vi "Main_backup.vi"() -> ()   [LabVIEW 2019]
uses:
  <vilib>/ptbypt/NI_PtbyPt.lvlib
panel:
  in  "low cutoff freq y":dbl=0.125 format="%0.3f"
  out "Filtered Correction y":dbl format="%0.2f"
  out "Filtered Correction x":dbl format="%0.2f"
  in  "low cutoff freq x":dbl=0.1 format="%#_13g"
  out "Filtered Correction y":dbl(graph)
  out "Filtered Correction x":dbl(graph)
  out "Height":dbl
  out "Motor 4 Correction":dbl
  out "Motor 3 Correction":dbl
  out "Motor 2 Correction":dbl
  out "Motor 1 Correction":dbl
  out "error out":errorcluster
  out "error out 2":errorcluster
  out "error out 5":errorcluster
  out "error out 6":errorcluster
  in  "PID Gains":T1={"Proportional Gain (Kc)"=0.8, "Integral Gain"=0.0, "Derivative Gain"=0.0}
  in  "Initial Motor Power":dbl
  in  "Boolean":bool
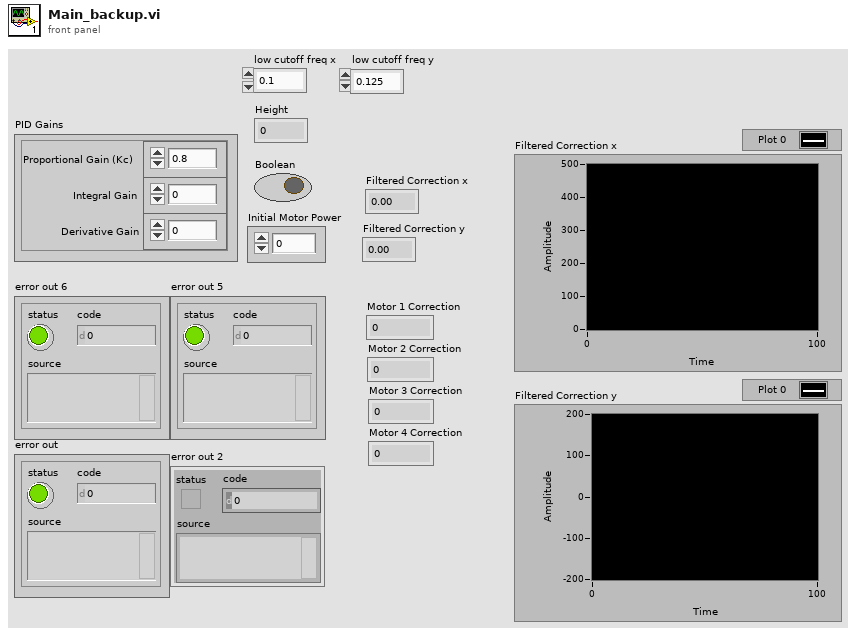
[diagram p1: front panel]
types:
  T1 = cluster{"Proportional Gain (Kc)":dbl, "Integral Gain":dbl, "Derivative Gain":dbl}
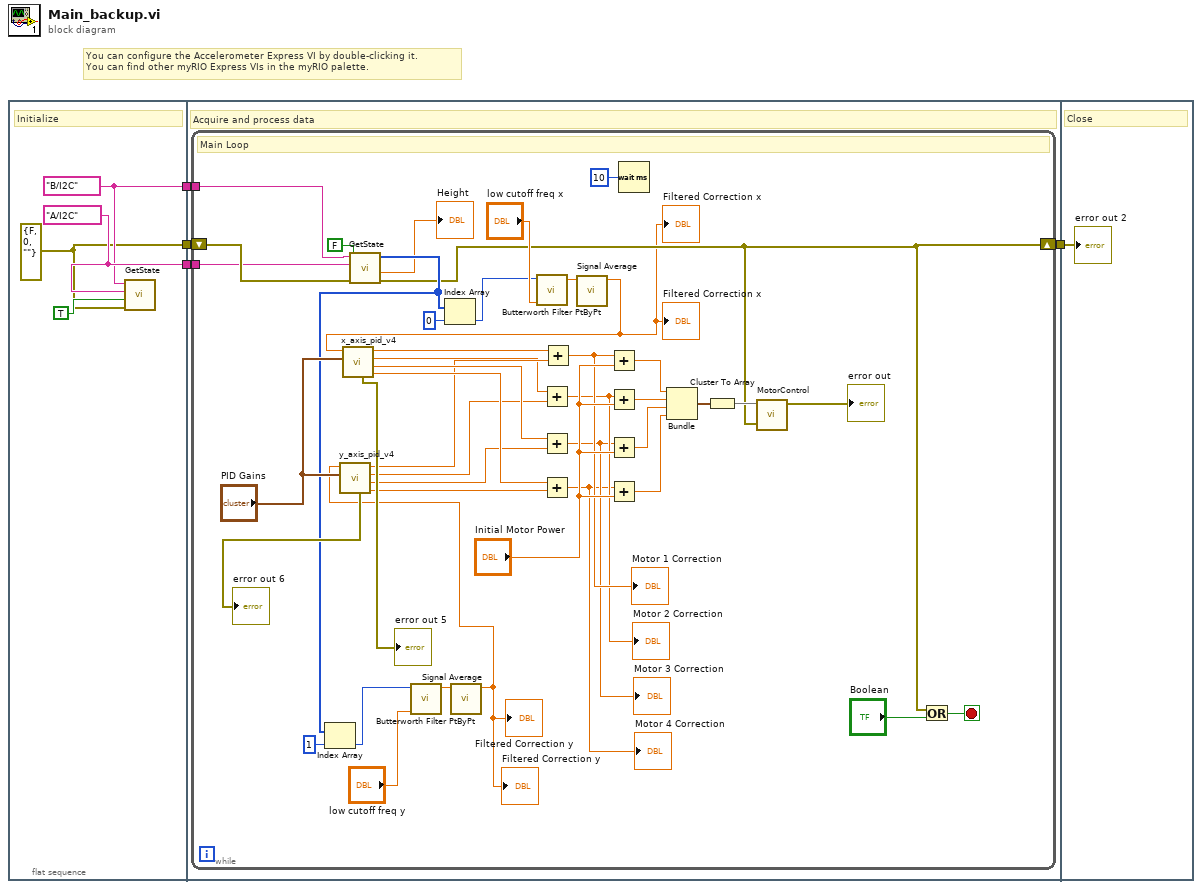
[diagram p0: block diagram]
diagram:
  # "You can configure the Accelerometer Express VI by double-clicking it.\nYou can find other myRIO Express VIs in the myRIO palette."
  n1 = flat-sequence {
    tunnel: [w7] -> w4
    tunnel: [w8] -> w3
    tunnel: [w5] -> w2
    tunnel: [w12] -> w1
    tunnel: w4 -> [w11]
    tunnel: w3 -> [w10]
    tunnel: w2 -> [w9]
    tunnel: w1 -> [w56]
    frame #0 {
      w8 = tag "A/I2C" ("IMU Channel")
      w7 = tag "B/I2C" ("LIDAR Channel")
      w5 = errorcluster {"status"=FALSE, "code"=0, "source"=""} ("error in (no error)")
      # "Initialize"
      n2 = call "GetState.vi"("error in (no error)"=w5, "Calibrate?"=TRUE, "IMU Channel"=w8, "LIDAR Channel"=w7) -> ()  [unwired: 2 in, 4 out]
    }
    frame #1 {
      # "Acquire and process data"
      n3 = while {
        shift-right: [w23] -> w12
        shift-left: w9 -> [w54]
        tunnel: w11 -> [w52]
        tunnel: w10 -> [w51]
        stop <- w55 stop-if-true
        # "Main Loop"
        n4 = call "GetState.vi"("error in (no error)"=w54, "Calibrate?"=FALSE, "IMU Channel"=w51, "LIDAR Channel"=w52) -> ("error out"=w23:errorcluster, "Height"=→"Height":dbl, "imu accel"=w34:i16[])  [unwired: 2 in, 1 out]
        n5 = Index Array(array=w34, index=1) -> (element=w35:i16)
        n6 = call <vilib>:"Butterworth Filter PtByPt.vi"("low cutoff freq: fl"="low cutoff freq y", "x"=w35) -> ("Filtered x"=w14:dbl)  [unwired: 7 in, 1 out]
        n7 = Index Array(array=w34, index=0) -> (element=w37:i16)
        n8 = call "Signal Average.vi"("Filtered Correction"=w14) -> ("Average Signal"=w13:dbl)  [unwired: 10 in]
        "Filtered Correction y" <- w13
        "Filtered Correction y" <- w13
        n9 = call "y_axis_pid_v4.vi"("PID Gains"="PID Gains", "Y In"=w13) -> ("Motor 4"=w41:dbl, "Motor 3"=w42:dbl, "Motor 2"=w43:dbl, "Motor 1"=w25:dbl, "error out"=→"error out 6":errorcluster)  [unwired: 5 in]
        n10 = call <vilib>:"Butterworth Filter PtByPt.vi"("low cutoff freq: fl"="low cutoff freq x", "x"=w37) -> ("Filtered x"=w16:dbl)  [unwired: 7 in, 1 out]
        n11 = call "Signal Average.vi"("Filtered Correction"=w16) -> ("Average Signal"=w17:dbl)  [unwired: 10 in]
        "Filtered Correction x" <- w17
        "Filtered Correction x" <- w17
        n12 = call "x_axis_pid_v4.vi"("PID Gains"="PID Gains", "X In"=w17) -> ("Motor 4"=w44:dbl, "Motor 3"=w45:dbl, "Motor 2"=w24:dbl, "Motor 1"=w46:dbl, "error out"=→"error out 5":errorcluster)  [unwired: 5 in]
        n13 = Add(x=w24, y=w43) -> (x+y=w21:dbl)
        "Motor 2 Correction" <- w21
        n14 = Add(x=w45, y=w42) -> (x+y=w20:dbl)
        "Motor 3 Correction" <- w20
        n15 = Add(x=w44, y=w41) -> (x+y=w19:dbl)
        "Motor 4 Correction" <- w19
        n16 = Add(x=w46, y=w25) -> (x+y=w22:dbl)
        "Motor 1 Correction" <- w22
        n17 = Add(x=w22, y="Initial Motor Power") -> (x+y=w31:dbl)
        n18 = Add(x=w21, y="Initial Motor Power") -> (x+y=w30:dbl)
        n19 = Add(x=w20, y="Initial Motor Power") -> (x+y=w29:dbl)
        n20 = Add(x=w19, y="Initial Motor Power") -> (x+y=w28:dbl)
        n21 = Wait (ms)(milliseconds to wait=u32 10) -> ()  [unwired: 1 out]
        n22 = Bundle(w31, w30, w29, w28) -> (w27:cluster{dbl, dbl, dbl, dbl})  [unwired: 1 in]
        n23 = Cluster To Array(cluster=w27) -> (array=w26:dbl[])
        n24 = call "MotorControl.vi"("error in (no error)"=w23, "Array"=w26) -> ("error out"=→"error out":errorcluster)  [unwired: 9 in]
        n25 = Or(x=w23, y="Boolean") -> (x .or. y?=w55:bool)
      }
    }
    frame #2 {
      # "Close"
      "error out 2" <- w56
    }
  }
